vi "S4GUI.vi"() -> ()   [LabVIEW 2018] (continued)
        n3369 = call "Next State.vi"("error in (no error)"=w8277, "New_State"=10, "State Machine in"=w8280) -> ("error out"=w8276:errorcluster, "State Machine out"=w8275:refnum<class "State Machine.lvclass">)  [unwired: 7 in]
        n3370 = call-dynamic "Write State Machine.vi"("error in (no error)"=w8276, "State Machine.lvclass"=w8275, "Device in"=w8274) -> ("error out"=w8271:errorcluster, "Device out"=w8273:refnum<class "Opt_Selector.lvclass">)  [unwired: 7 in]
        n3371 = call "Write ASEL.vi"("error in (no error)"=w8271, "Opt_Selector.lvclass"=w8273, "Instrument in"=w8272) -> ("error out"=w8268:errorcluster, "Instrument out"=w8270:refnum<class "Instrument.lvclass">)  [unwired: 7 in]
        n3372 = call "Write Instrument.lvclass.vi"("error in (no error)"=w8268, "Instrument.lvclass"=w8270, "S4ACS_GUI in"=w8269) -> ("error out"=w8267:errorcluster, "S4ACS_GUI out"=w8266:refnum<class "S4GUI.lvclass">)  [unwired: 7 in]
      }
      event "ASEL_init": Value Change {
        n3373 = event-data() -> ()  [unwired: 1 in, 4 out]
        n3374 = call "Read Instrument.lvclass.vi"("error in (no error)"=w8304, "S4ACS_GUI in"=w8305) -> ("error out"=w8302:errorcluster, "Instrument.lvclass"=w8303:refnum<class "Instrument.lvclass">, "S4ACS_GUI out"=w8289:refnum<class "S4GUI.lvclass">)  [unwired: 7 in]
        n3375 = call "Read ASEL.vi"("error in (no error)"=w8302, "Instrument in"=w8303) -> ("error out"=w8298:errorcluster, "Opt_Selector.lvclass"=w8301:refnum<class "Opt_Selector.lvclass">, "Instrument out"=w8292:refnum<class "Instrument.lvclass">)  [unwired: 7 in]
        n3376 = call-dynamic "Read State Machine.vi"("error in (no error)"=w8298, "Device in"=w8301) -> ("error out"=w8297:errorcluster, "State Machine.lvclass"=w8300:refnum<class "State Machine.lvclass">, "Device out"=w8294:refnum<class "Opt_Selector.lvclass">)  [unwired: 7 in]
        n3377 = call "Next State.vi"("error in (no error)"=w8297, "New_State"=30, "State Machine in"=w8300) -> ("error out"=w8296:errorcluster, "State Machine out"=w8295:refnum<class "State Machine.lvclass">)  [unwired: 7 in]
        n3378 = call-dynamic "Write State Machine.vi"("error in (no error)"=w8296, "State Machine.lvclass"=w8295, "Device in"=w8294) -> ("error out"=w8291:errorcluster, "Device out"=w8293:refnum<class "Opt_Selector.lvclass">)  [unwired: 7 in]
        n3379 = call "Write ASEL.vi"("error in (no error)"=w8291, "Opt_Selector.lvclass"=w8293, "Instrument in"=w8292) -> ("error out"=w8288:errorcluster, "Instrument out"=w8290:refnum<class "Instrument.lvclass">)  [unwired: 7 in]
        n3380 = call "Write Instrument.lvclass.vi"("error in (no error)"=w8288, "Instrument.lvclass"=w8290, "S4ACS_GUI in"=w8289) -> ("error out"=w8287:errorcluster, "S4ACS_GUI out"=w8286:refnum<class "S4GUI.lvclass">)  [unwired: 7 in]
      }
    }
    n3381 = local read "P0"() -> (w47:bool)
    n3382 = local write "P0"(w47) -> ()
    n3383 = flat-sequence {
      tunnel: w55 -> [w75]
      tunnel: w53 -> [w73]
      tunnel: [w75] -> w52
      tunnel: [w71] -> w51
      tunnel: [w70] -> w50
      tunnel: [w78] -> w54
      tunnel: w52 -> [w78]
      tunnel: w51 -> [w77]
      tunnel: w50 -> [w76]
      frame #0 {
        n3384 = Tick Count (ms)() -> (millisecond timer value=w74:u32)
        n3385 = local read "loop max(ms)"() -> (w69:u32)
        n3386 = Subtract(x=w74, y=w73) -> (x-y=w71:u32)
        n3387 = Greater?(x=w71, y=w69) -> (0:w72:bool)
        n3388 = Select(t=w71, s=w72, f=w69) -> (s? t:f=w70:u32)
      }
      frame #1 {
        "loop time(ms)" <- w77
        "loop max(ms)" <- w76
      }
    }
  }
  n3389 = stacked-sequence "INTERFACE" {
    frame #0 {
    }
    frame #1 {
    }
    frame #2 {
    }
    frame #3 {
    }
    frame #4 {
    }
    frame #5 {
    }
    frame #6 {
    }
    frame #7 {
    }
  }
  n3390 = disable-structure shown="Enabled" {
    frame Disabled {
      n3391 = Unbundle By Name() -> ("CALW State"=w8309:i32, "ASEL State"=w8308:i32, "GMIR State"=w8307:i32, "GFOC State"=w8306:i32)  [unwired: 1 in, 2 out]
      n3392 = Not Equal To 0?(x=w8309) -> ()  [unwired: 1 out]
      n3393 = Not Equal To 0?(x=w8308) -> ()  [unwired: 1 out]
      n3394 = Not Equal To 0?(x=w8307) -> ()  [unwired: 1 out]
      n3395 = Not Equal To 0?(x=w8306) -> ()  [unwired: 1 out]
    }
    frame Enabled {
    }
  }
  n3396 = call-dynamic "End.vi"("S4ACS_GUI in"=w27) -> ("error out"=→"error out":errorcluster)  [unwired: 9 in, 1 out]
